vi "Coincidence_rs232(BEREA)WDAQ.vi"() -> ()   [LabVIEW 2017]
doc: "This is the program you use to run one of 4 different experiments:\n 1) Simply measuring coincidences between two beams.\n 2) Measuring g(2)(0) for 2-beams using 3-detectors.\n 3) Measuring single photon interference patterns (and simultaneously g(2)(0) for 2-beams using 3-detectors).\n 4) Measuring g(2)(0) for 1-beam using 2-detectors.\nNote that g(2) is calculated differently depending on whether you're making 3-detector or 2-detector measurements. See details in the description of the \"g(2) Measurements\" parameter.\nThis vi was specifically written for the Altera DE2 counter. Data streams to the computer from the DE2 over the RS232 serial port.\nThe program does not record data to a file right away, but displays the counters in real time so that you can align things. \nOnce everything is aligned and the parameters are set, you press the \"Take Data\" button. This transfers control to another program which records a data set and saves it to a file. \nNote that there is one control: \"NewStep?\" that tells the computer what hardware you have present in your experiment. This control is not visible normally. It located below the \"Data Taking Parameters\", so you'll need to scroll the window down to access it. This control is only read once at the beginning of execution--so it must be properly set BEFORE you run the program.\nThe \"NewStep?\" control tells the computer whether or not you have a NewStep stepper motor attached to your computer to control phase adjustments of the interferometer. This control is useful so that the computer won't try to communicate with an instrument you don't have, causing a hang-up. By default \"NewStep?\" is set to \"No\"--if you do have a NewStep, you'll want to change the default to \"Yes\". For more info see the description of this control below.\nFor interference measurements, a Newport NewStep actuator (inexpensive stepper motor) is used to tilt a beam displacing polarizer to adjust the phase of a polarization interferometer. This actuator is controlled by a NewStep controller, connected to a serial port of the computer with an RS-485 to RS-232 converter. If you do not have this controller, set the \"NewStep?\" parameter to \"No\".\nSignals that should be selected on the DE2 for the coincidence counters:\n______________________________________\nA (Counter 0)\nB (Counter 1)\nA' (Counter 2) - unused by this vi\nB' (Counter 3)\nAB (Counter 4)\nABB' (Counter 5) - used for 3-detector g2 measurements (and interference)\nAB' (Counter 6)\nBB' (Counter 7) - used for 2-detector g2 measurements\n__________________________________________________\nNote that for the coincidence experiment, only 3 counters are used: A, B, and AB. For the other 3 experiments, 7 counters are used. \nOn startup, the program initializes the counters.\nAfter initialization the program simply loops and displays the counts in a given time window (determined by the \"Update Period\" control in the upper left.) This is useful for tweaking the alignment and adjusting parameters. \nNothing is written to disk until the parameters are chosen and the \"Take Data\" button is pressed. This loads a second VI that records and saves data to disk. Parameters for this data acquisition phase are set in the \"Data Taking Parameters\" box.\nWhen performing an interference experiment, the stepper motor will automatically adjust the tilt of the beam displacing prism, changing the phase. \nHelp for each of the controls and indicators can be obtained from the Contextual Help window <cntrl - H> by mousing over each control or indicator. Full documentation for each control and indicator can be obtained by printing using: File>Print>Custom, and then checking \"All controls\" and \"Descriptions\"."
uses:
  <vilib>/Utility/file.llb/Write Delimited Spreadsheet (DBL).vi
panel:
  out "Current Value of \nDAC  input":u16
  in  "?":T1(tab)
  in  "Tab Control":enum32{"Data Acquisition"}(tab)
  in  "Update Period (Data Run)":dbl=1.0 min=0.1 max=1000.0 step=0.1 format="%.1f"
  in  "Range to scan (±)":u32=100
  in  "Center stepper position\n(µsteps)":u32=26000 min=10000 max=50000 step=1
  in  "Number of points":i32=3
  in  "Take Data":bool
  in  "g(2) Measurements":enum32{"Page 1", "Page 2"}(tab)
  in  "Clear Buffer":bool
  out "Buffer size":u32=60
  out "g(2)":dbl=nan format="%.3f"
  in  "Max Buffer":u32=60
  out "g(2) Std. Dev.":dbl=nan format="%.3f"
  out "Ave.g(2)":dbl=nan format="%.3f"
  in  "Experimental\n Setup":i32(knob) min=0 max=3 step=1 scale=0.0..3.0
  in  "Counter Port":refnum<visa-resource-name>="COM3"
  in  "Update Period":dbl=0.30000000000000004 min=0.1 max=200.0 step=0.1 format="%.1f"
  out "Error Out":errorcluster
  in  "ABB' Coincidence\n window":dbl=4.76 caption="ABB' Coincidence \nWindow (ns)" min=0.1 max=500000.0 step=0.01 format="%.2f"
  in  "2D window stdev":dbl=0.03 caption="+" min=0.0 max=500000.0 step=0.001 format="%.2f"
  in  "BB' Coincidence\n window":dbl=7.39 caption="BB' Coincidence \nWindow (ns)" min=0.1 max=500000.0 step=0.01 format="%.2f"
  in  "Set DAC to 0":bool
  in  "Ramp DAC":bool
  in  "Save Data":bool
  out "Expt ind":i32
  in  "graphs 2":enum32{"B & B'", "BB'", "g(2)(0)"}(tab)
  out "BB'":u32(graph)
  out "g2":dbl(graph)=nan
  out "BB'":u32(slide) scale=0.0..3500.0 scale format="%_2p"
  in  "graphs":T2(tab)
  out "B & B'":cluster{u32, u32}(graph)
  out "AB & AB'":cluster{u32, u32}(graph)
  out "g2":dbl(graph)=nan
  out "BB' vs Voltage":cluster{u32, u32, u32}(graph)
  in  "?":enum32{"Stepper Control"}(tab)
  out "ABB'":u32(slide) scale=0.0..30.0 scale format="%_2p"
  out "B & B'":u32[](array[slide]) scale=0.0..250000.0 scale format="%_2p"
  out "A":u32(slide) scale=0.0..500000.0 scale format="%_2p"
  in  "stop":bool
  out "AB &  AB'":u32[](array[slide]) scale=0.0..20000.0 scale format="%_2p"
  # "AB'"
  # "AB"
  # "B"
  # "B'"
  # "Data Taking Parameters"
  # "(must be a \nmultiple of 0.1s)"
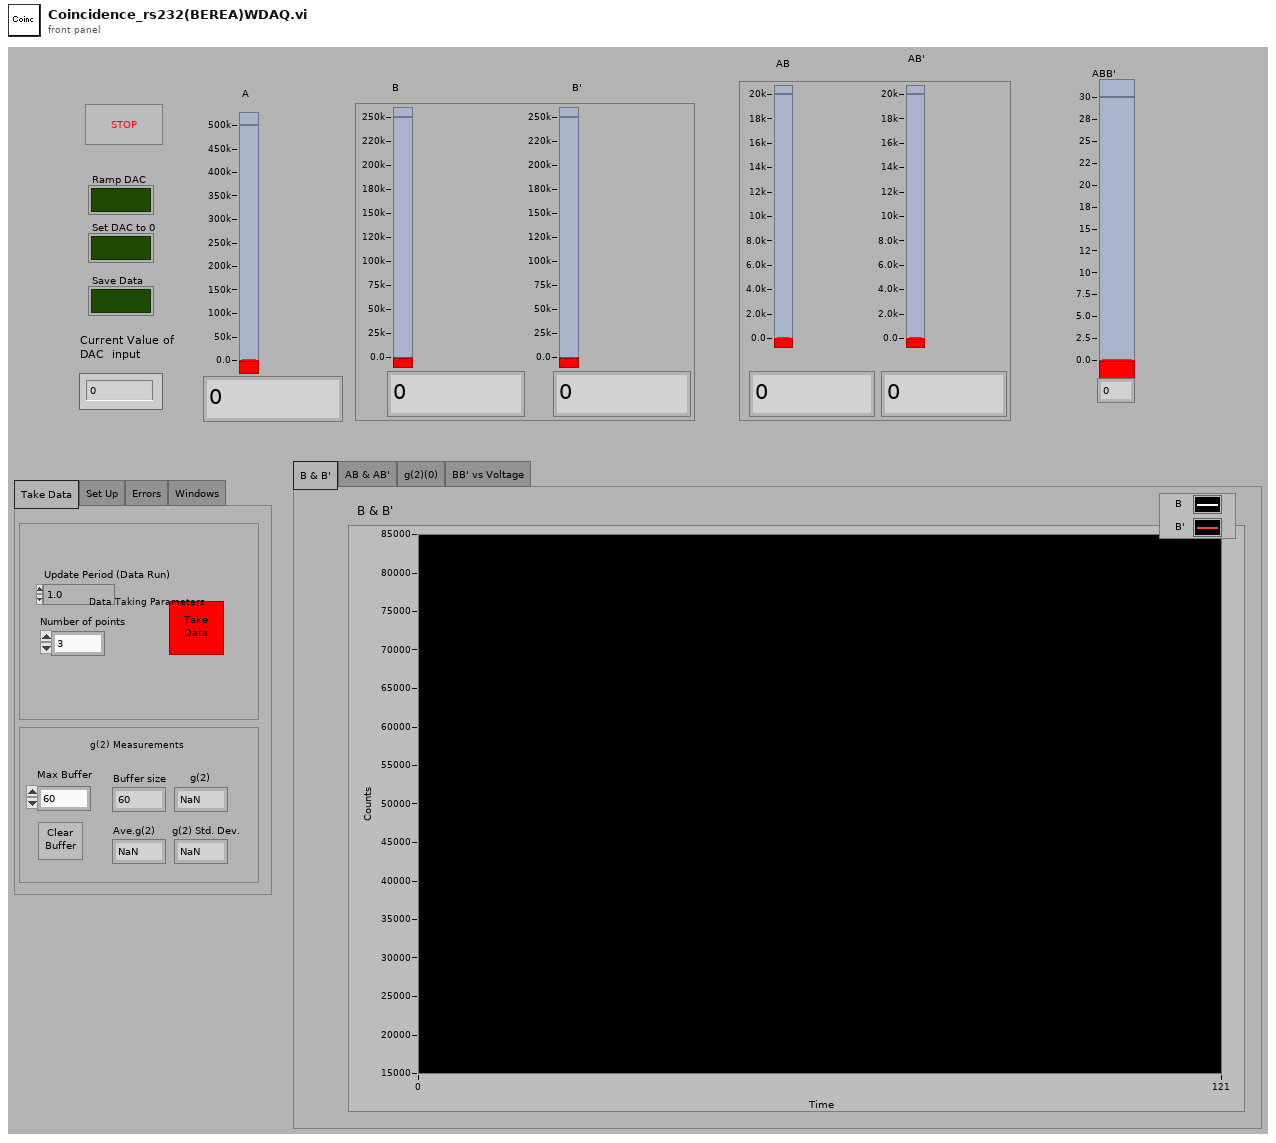
[diagram p1: front panel]
types:
  T1 = enum32{"Take Data", "Set Up", "Errors", "Windows"}
  T2 = enum32{"B & B'", "AB & AB'", "g(2)(0)", "BB' vs Voltage"}
  T3 = cluster{"BB' Coincidence\n window":dbl, "2D window stdev":dbl, "ABB' Coincidence\n window":dbl}
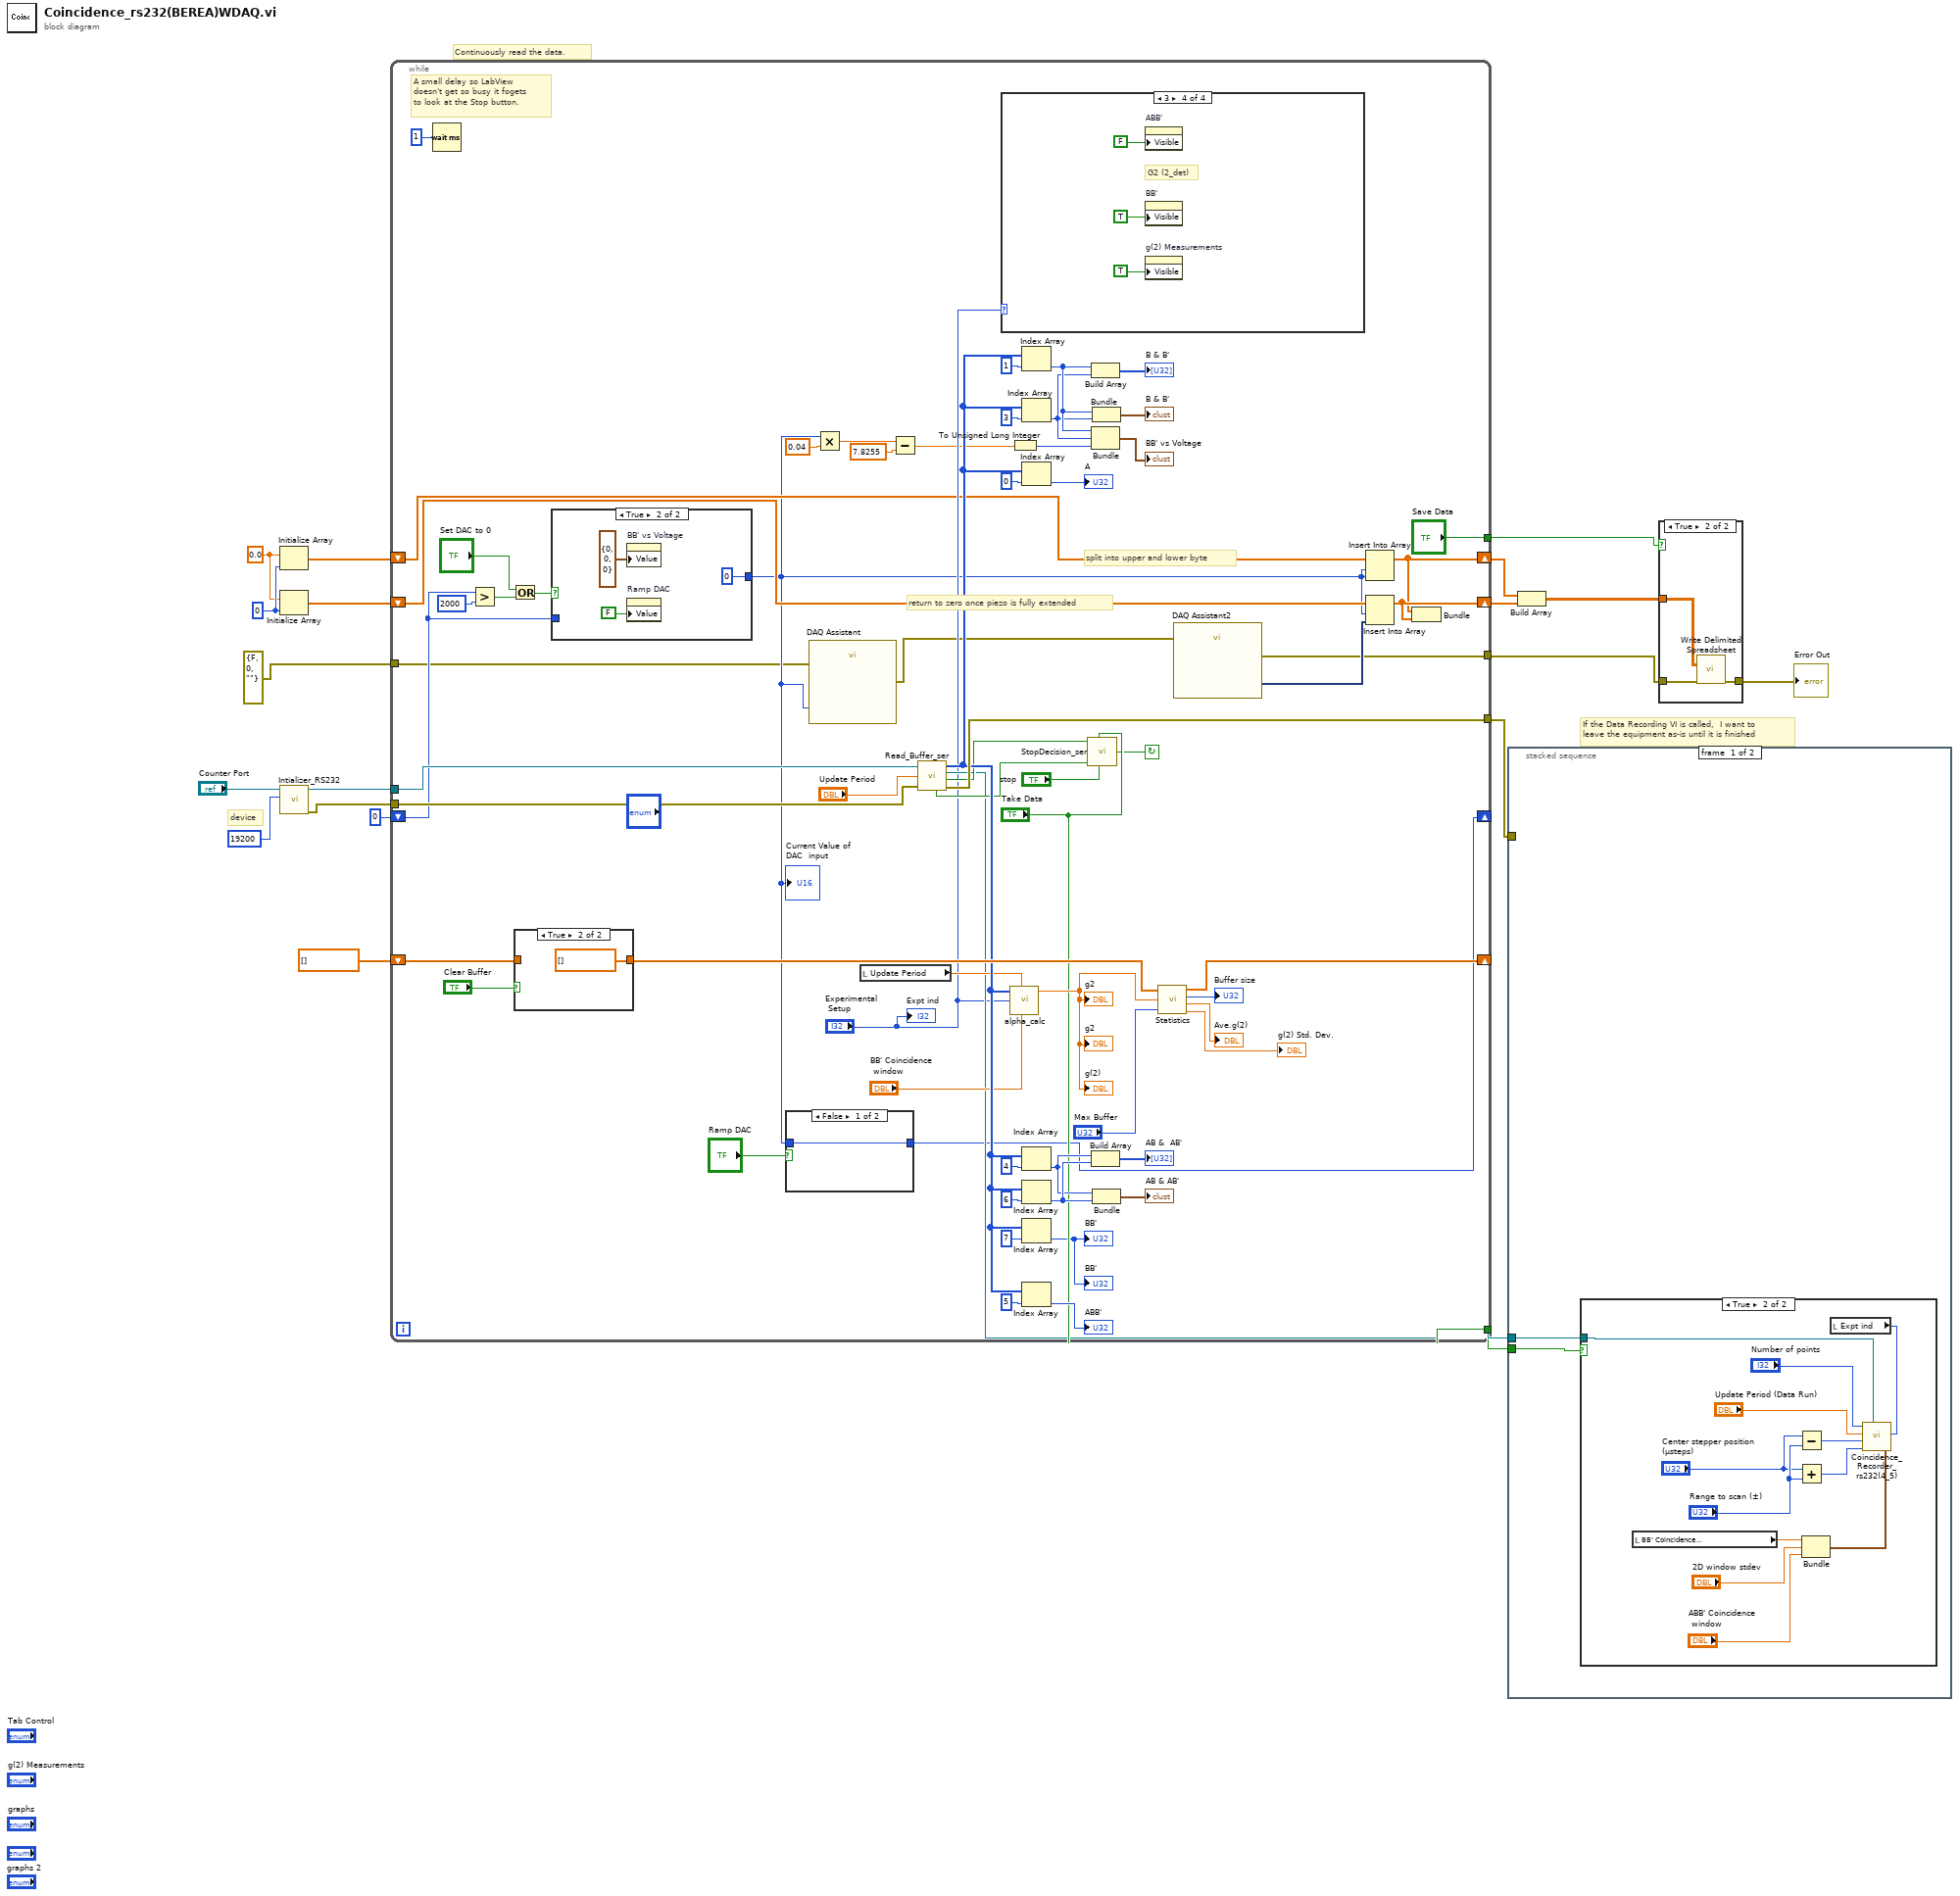
[diagram p0: block diagram]
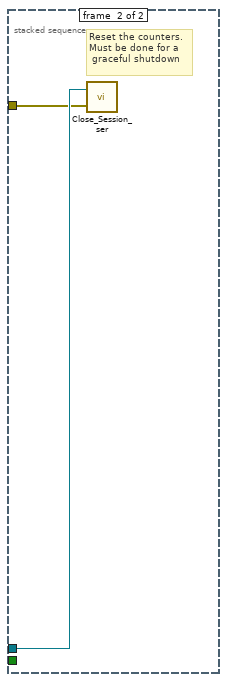
[diagram p4: hidden frame]
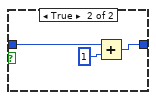
[diagram p5: hidden frame]
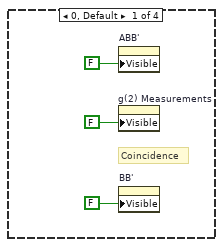
[diagram p8: hidden frame]
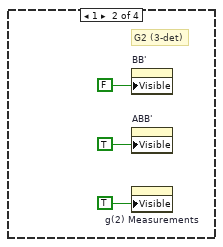
[diagram p9: hidden frame]
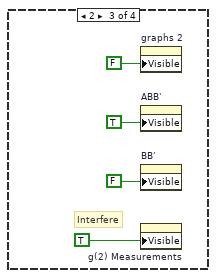
[diagram p10: hidden frame]
diagram:
  w11 = 0.0 ("element")
  w12 = 0 ("dimension size")
  # "If the Data Recording VI is called,  I want to \nleave the equipment as-is until it is finished"
  # "Continuously read the data."
  # "device"
  n1 = Initialize Array(w11, w12) -> (w8:dbl[])
  n2 = Initialize Array(w11, w12) -> (w7:dbl[])
  n3 = call "Intializer_RS232.vi"("baud rate"=u32 19200 ("device"), "Counter Port"="Counter Port") -> ("error out"=w19:errorcluster, "Counter port out"=w18:refnum<visa-resource-name>)  [unwired: 4 in]
  n4 = while {
    tunnel: w18 -> [w49]
    tunnel: w19 -> [w81]
    tunnel: [w80] -> w14
    tunnel: [w48] -> w16
    shift-right: [w66] -> _
    shift-left: dbl[] [] ("Output Array") -> [w68]
    tunnel: ["Take Data"] -> w15
    tunnel: ["Save Data"] -> w4
    shift-right: [w40] -> _
    shift-left: 0 -> [w39]
    shift-right: [w37] -> w5
    shift-left: w7 -> [w46]
    shift-right: [w36] -> w6
    shift-left: w8 -> [w38]
    tunnel: errorcluster {"status"=FALSE, "code"=0, "source"=""} ("error in") -> [w24]
    tunnel: [w21] -> w1
    stop <- w51 continue-if-true
    # "return to zero once piezo is fully extended"
    # "split into upper and lower byte"
    # "A small delay so LabView\ndoesn't get so busy it fogets\nto look at the Stop button."
    n5 = Wait (ms)(milliseconds to wait=u32 1) -> ()  [unwired: 1 out]
    n6 = Greater?(x=w39, y=2000) -> (0:w33:bool)
    n7 = Or(x="Set DAC to 0", y=w33) -> (x .or. y?=w32:bool)
    n8 = case shown="True" "Clear Buffer" {
      tunnel: w68 -> [w94 _]
      tunnel: [w94 dbl[] [] ("Output Array")] -> w67
      frame False {
      }
      frame True {
      }
    }
    n9 = case shown="True" w32 {
      tunnel: [w90 0] -> w25
      tunnel: w39 -> [w90 _]
      frame False {
      }
      frame True {
        n10 = property on="BB' vs Voltage" class="WFChart (strict)"("Value"=cluster{u32, u32, u32} {0, 0, 0} ("BB' vs Voltage")) -> ()  [unwired: 2 in, 2 out]
        n11 = property on="Ramp DAC" class="Bool (strict)"("Value"=FALSE ("Boolean")) -> ()  [unwired: 2 in, 2 out]
      }
    }
    "Current Value of \nDAC  input" <- w25
    n12 = case shown="False" "Ramp DAC" {
      tunnel: w25 -> [w86 w88]
      tunnel: [w86 w87] -> w40
      frame False {
      }
      frame True {
        n13 = Add(x=w88, y=1) -> (x+y=w87:i32)
      }
    }
    n14 = call "DAQ Assistant"("data"=w25, "error in"=w24) -> ("error out"=w22:errorcluster)  [unwired: 16 in, 1 out]
    n15 = Multiply(x=w25, y=0.04) -> (x*y=w44:dbl)
    n16 = local read "Update Period"() -> (w56:dbl)
    n17 = Subtract(x=w44, y=7.8255) -> (x-y=w30:dbl)
    n18 = call "Read_Buffer_ser.vi"("error in"=w81, "Update Period (s)"="Update Period", "Counter Port"=w49) -> ("error out"=w80:errorcluster, "status"=w54:bool, "Finished"=w55:bool, "Counter port out"=w48:refnum<visa-resource-name>, "The actual numbers"=w58:u32[])  [unwired: 1 in]
    n19 = case shown="3" "Experimental\n Setup" {
      frame 0, Default {
        # "Coincidence"
        n20 = property on="ABB'" class="Slide (strict)"("Visible"=FALSE) -> ()  [unwired: 2 in, 2 out]
        n21 = property on="g(2) Measurements" class="TabCtl (strict)"("Visible"=FALSE) -> ()  [unwired: 2 in, 2 out]
        n22 = property on="BB'" class="Slide (strict)"("Visible"=FALSE) -> ()  [unwired: 2 in, 2 out]
      }
      frame 1 {
        # "G2 (3-det)"
        n23 = property on="BB'" class="Slide (strict)"("Visible"=FALSE) -> ()  [unwired: 2 in, 2 out]
        n24 = property on="ABB'" class="Slide (strict)"("Visible"=TRUE) -> ()  [unwired: 2 in, 2 out]
        n25 = property on="g(2) Measurements" class="TabCtl (strict)"("Visible"=TRUE) -> ()  [unwired: 2 in, 2 out]
      }
      frame 2 {
        # "Interfere"
        n26 = property on="graphs 2" class="TabCtl (strict)"("Visible"=FALSE) -> ()  [unwired: 2 in, 2 out]
        n27 = property on="ABB'" class="Slide (strict)"("Visible"=TRUE) -> ()  [unwired: 2 in, 2 out]
        n28 = property on="BB'" class="Slide (strict)"("Visible"=FALSE) -> ()  [unwired: 2 in, 2 out]
        n29 = property on="g(2) Measurements" class="TabCtl (strict)"("Visible"=TRUE) -> ()  [unwired: 2 in, 2 out]
      }
      frame 3 {
        # "G2 (2_det)"
        n30 = property on="ABB'" class="Slide (strict)"("Visible"=FALSE) -> ()  [unwired: 2 in, 2 out]
        n31 = property on="BB'" class="Slide (strict)"("Visible"=TRUE) -> ()  [unwired: 2 in, 2 out]
        n32 = property on="g(2) Measurements" class="TabCtl (strict)"("Visible"=TRUE) -> ()  [unwired: 2 in, 2 out]
      }
    }
    n33 = call "alpha_calc.vi"("data"=w58, "Update Period"=w56, "Experiment"="Experimental\n Setup", "Coincidence\n window"="BB' Coincidence\n window") -> ("Alpha"=w59:dbl)  [unwired: 3 in]
    "g(2)" <- w59
    "g2" <- w59
    "g2" <- w59
    n34 = To Unsigned Long Integer(number=w30) -> (unsigned 32bit integer=w29:u32)
    n35 = Index Array(array=w58, index=1) -> (element=w27:u32)
    n36 = Index Array(array=w58, index=3) -> (element=w26:u32)
    n37 = Index Array(array=w58, index=0) -> (element=→"A":u32)
    n38 = Index Array(array=w58, index=4) -> (element=w71:u32)
    n39 = Index Array(array=w58, index=6) -> (element=w72:u32)
    n40 = Index Array(array=w58, index=7) -> (element=→"BB'" →"BB'":u32)
    n41 = Index Array(array=w58, index=5) -> (element=→"ABB'":u32)
    n42 = call "StopDecision_ser.vi"("Stop Button"="stop", "Take Data Button"="Take Data", "STATUS"=w54, "Finished? 1"=w55) -> ("To \"Continue if true\""=w51:bool)  [unwired: 2 in]
    n43 = Build Array(w27, w26) -> (→"B & B'":u32[])
    n44 = Bundle(w27, w26, w29) -> (→"BB' vs Voltage":cluster{u32, u32, u32})  [unwired: 1 in]
    n45 = Build Array(w71, w72) -> (→"AB &  AB'":u32[])
    n46 = Bundle(w27, w26) -> (→"B & B'":cluster{u32, u32})  [unwired: 1 in]
    n47 = Bundle(w71, w72) -> (→"AB & AB'":cluster{u32, u32})  [unwired: 1 in]
    n48 = call "Statistics.vi"("Input Array"=w67, "Array element"=w59, "Max. Array Size"="Max Buffer") -> ("Output Array"=w66:dbl[], "Array size"=→"Buffer size":u32, "Mean"=→"Ave.g(2)":dbl, "Std. Dev."=→"g(2) Std. Dev.":dbl)
    n49 = call "DAQ Assistant2"("error in"=w22) -> ("data"=w23:dynamicdata, "error out"=w21:errorcluster)  [unwired: 16 in, 1 out]
    n50 = Insert Into Array(array=w38, index=w25, new element=w25) -> (w36:dbl[])
    n51 = Insert Into Array(array=w46, index=w25, new element=w23) -> (w37:dbl[])
    n52 = Bundle(w36, w37) -> ()  [unwired: 1 in, 1 out]
    "Expt ind" <- "Experimental\n Setup"
  }
  n53 = stacked-sequence {
    tunnel: w16 -> [w110 w124]
    tunnel: w15 -> [w109 _]
    tunnel: w14 -> [_ w123]
    frame #0 {
      n54 = case shown="True" w109 {
        tunnel: w110 -> [_ w120]
        frame False {
        }
        frame True {
          n55 = local read "BB' Coincidence\n window"() -> (w114:dbl)
          n56 = Subtract(x="Center stepper position\n(µsteps)", y="Range to scan (±)") -> (x-y=w119:u32)
          n57 = Add(x="Center stepper position\n(µsteps)", y="Range to scan (±)") -> (x+y=w118:u32)
          n58 = Bundle("BB' Coincidence\n window"=w114, "2D window stdev"="2D window stdev", "ABB' Coincidence\n window"="ABB' Coincidence\n window") -> (w113:T3)  [unwired: 1 in]
          n59 = local read "Expt ind"() -> (w115:i32)
          n60 = call "Coincidence_Recorder_rs232(4_5).vi"("Coincidence times"=w113, "Experiment"=w115, "Counter Port"=w120, "End stepper position"=w118, "Starting stepper position"=w119, "Time per update (s)"="Update Period (Data Run)", "Number of points"="Number of points") -> ()  [unwired: 3 in]
        }
      }
    }
    frame #1 {
      # "Reset the counters.\nMust be done for a\n graceful shutdown"
      n61 = call "Close_Session_ser.vi"("error in (no error)"=w123, "Counter Port"=w124) -> ()  [unwired: 1 in]
    }
  }
  n62 = Build Array(w6, w5) -> (w9:dbl[][])
  n63 = case shown="True" w4 {
    tunnel: [w125 w128] -> w10
    tunnel: w1 -> [w125 w126]
    tunnel: w9 -> [_ w127]
    frame False {
    }
    frame True {
      n64 = call-poly <vilib>:"Write Delimited Spreadsheet.vi"("2D data"=w127, "error in (no error)"=w126) -> ("error out"=w128:errorcluster)  [unwired: 12 in, 1 out]
    }
  }
  "Error Out" <- w10
